vi "WriteTestItemInstruction.vi"() -> ()   [LabVIEW 2013]
panel:
  out "error out":errorcluster caption="错误输出"
  in  "error in":errorcluster caption="错误输入（无错误）"
  out "大小":i32
  out "输出数组":string[](array[string])
  out "连接的字符串":string
  out "ReportStrA":string
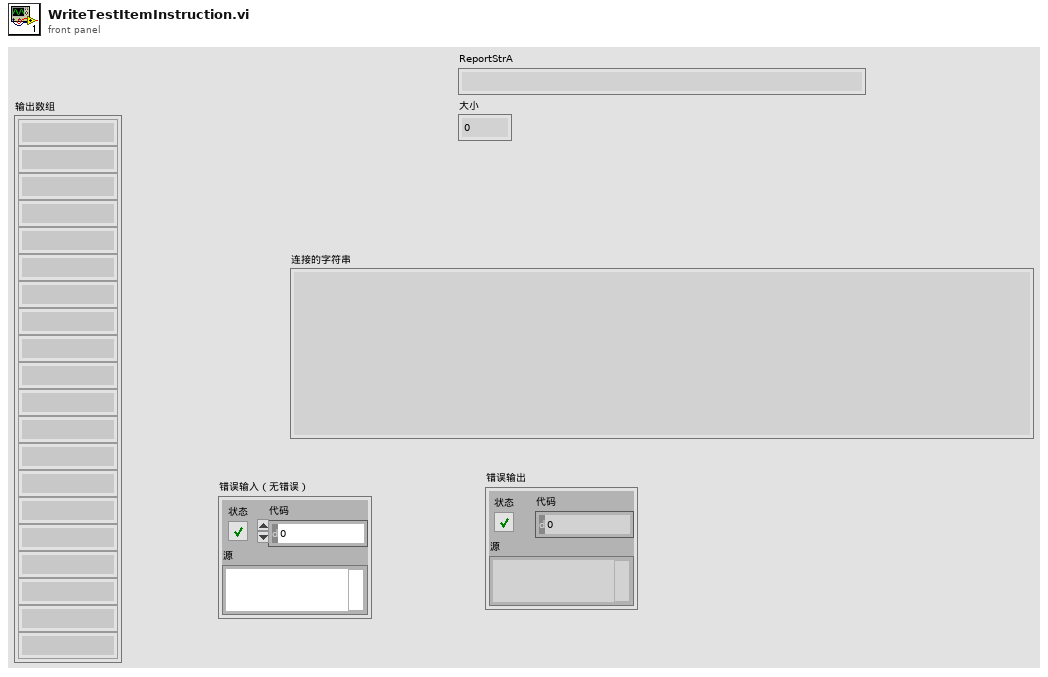
[diagram p1: front panel]
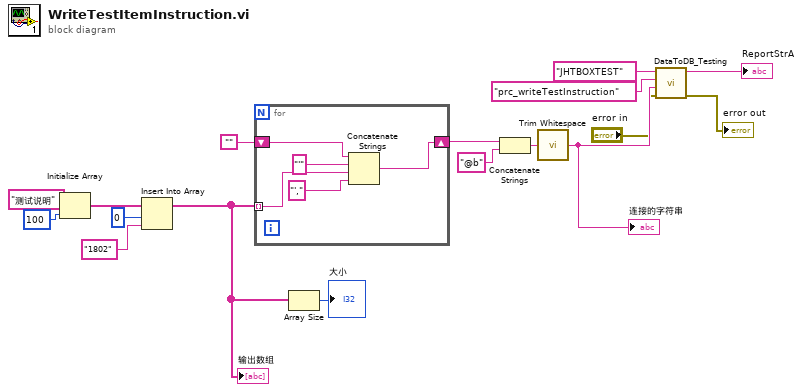
[diagram p0: block diagram]
diagram:
  n1 = Initialize Array("测试说明", 100 ("维数大小")) -> (w11:string[])
  n2 = Insert Into Array(array=w11, index=0 ("索引"), new element="1802") -> (w4:string[])
  "输出数组" <- w4
  n3 = for {
    shift-right: [w18] -> w8
    shift-left: "" -> [w22]
    tunnel: w4 -> [w19] mode=indexing
    n4 = Concatenate Strings(w22, "'", w19, "',") -> (w18:string)
  }
  n5 = Array Size(array=w4) -> (size(s)=→"大小":i32)
  n6 = Concatenate Strings(w8, "@b") -> (w6:string)
  n7 = call <vilib>:"Trim Whitespace.vi"("string"=w6) -> ("trimmed string"=w5:string)  [unwired: 1 in]
  "连接的字符串" <- w5
  n8 = call "DataToDB_Testing.vi"("error in (no error)"="error in", "all string"=w5, "Procedure name"="prc_writeTestInstruction", "DSN name"="JHTBOXTEST") -> ("error out"=→"error out":errorcluster, "ReportStrA"=→"ReportStrA":string)  [unwired: 6 in]
